vi "DAQ_PID_Actuator.vi"() -> ()   [LabVIEW 2019]
uses:
  <vilib>/Platform/TimedLoop/XDataNode/timing_clust.ctl
  <vilib>/Platform/TimedLoop/XDataNode/nitl_modes.ctl
  <vilib>/Platform/TimedLoop/XDataNode/wakeup.ctl
  <vilib>/Analysis/6fits.llb/Curve Fitting Criteria.ctl
  <vilib>/Analysis/3filter.llb/Filter Passband Type.ctl
  <vilib>/DAQmx/write.llb/DAQmx Write (Analog Wfm 1Chan NSamp).vi
  <vilib>/DAQmx/read.llb/DAQmx Read (Analog Wfm 1Chan NSamp).vi
  <vilib>/Analysis/baseanly.llb/Mean (DBL).vi
  <vilib>/Analysis/5stat.llb/RMS (DBL).vi
  <vilib>/DAQmx/create/channels.llb/DAQmx Create Channel (AO-Voltage-Basic).vi
  <vilib>/DAQmx/configure/timing.llb/DAQmx Timing (Sample Clock).vi
  <vilib>/DAQmx/miscellaneous.llb/DAQmx Fill In Error Info.vi
  <vilib>/DAQmx/create/channels.llb/DAQmx Create Channel (AI-Voltage-Basic).vi
  <vilib>/measure/mascope.llb/Amplitude and Levels 1 chan (obs).vi
  <vilib>/gmath/NumericalOptimization/Nonlinear Curve Fit LM formula string.vi
  <vilib>/platform/TimedLoop/XDataNode/XDataNode.xnode
  <vilib>/Analysis/NI_AALBase.lvlib
  <vilib>/Platform/TimedLoop/XDataNode/XDNodeRunTimeDep.lvlib
  <vilib>/gmath/NI_Gmath.lvlib
  <vilib>/Analysis/NI_AALPro.lvlib
  <vilib>/measure/NI_MABase.lvlib
  <vilib>/measure/NI_MAPro.lvlib
  <vilib>/ptbypt/NI_PtbyPt.lvlib
panel:
  out "Value":dbl min=-5.0 max=5.0 step=0.0001
  in  "Set Point Offset":dbl(slide) min=-5.0 max=5.0 step=0.0001 scale=-5.0..5.0
  in  "guessVoltage":dbl format="%#_13g"
  in  "PHASE":dbl format="%#_13g"
  in  "STOP":bool
  out "In Range?":bool=TRUE
  out "ELEMENT":dbl=0.9799129199459758
  in  "Ki":dbl=0.07
  in  "Kp":dbl=0.03
  out "SLOPE":dbl=-6.141102048812741
  out "OFFSET":dbl=1.2218182454508948
  out "Waveform Chart":dynamicdata(graph)=[{"t0"=timestamp(3637842565.871356 s since 1904-01-01), "dt"=1.0, "Y"=[2.0218377698329277]}, {"t0"=timestamp(3637842565.8663554 s since 1904-01-01), "dt"=1.0, "Y"=[0.25417959292529346]}, {"t0"=timestamp(3637842565.871356 s since 1904-01-01), "dt"=1.0, "Y"=[1.729518885187998]}, {"t0"=timestamp(3637842565.871356 s since 1904-01-01), "dt"=1.0, "Y"=[1.7676581769076343]}]
  in  "stop":bool
  out "Scanning":waveform(dbl)[](graph)=[{"t0"=timestamp(0 s since 1904-01-01), "dt"=0.000333325, "Y"=array[3000 elements]}, {"t0"=timestamp(0 s since 1904-01-01), "dt"=0.0003333333333333333, "Y"=array[3000 elements]}, {"t0"=timestamp(0 s since 1904-01-01), "dt"=0.000333325, "Y"=array[3000 elements], "attributes"=variant("NI_ChannelName"=variant(string "Filtered (Filtered)"), "NI_OriginalChannelName"=variant(string "Filtered"))}]
  in  "stop Lock":bool
  out "Locking":cluster{"Y":dbl[], "best nonlinear fit":dbl[]}[](graph)=[{"Y"=[1.5391142076213253], "best nonlinear fit"=[0.25417959292529346]}, {"Y"=array[214 elements], "best nonlinear fit"=array[214 elements]}, {"Y"=array[214 elements], "best nonlinear fit"=array[214 elements]}]
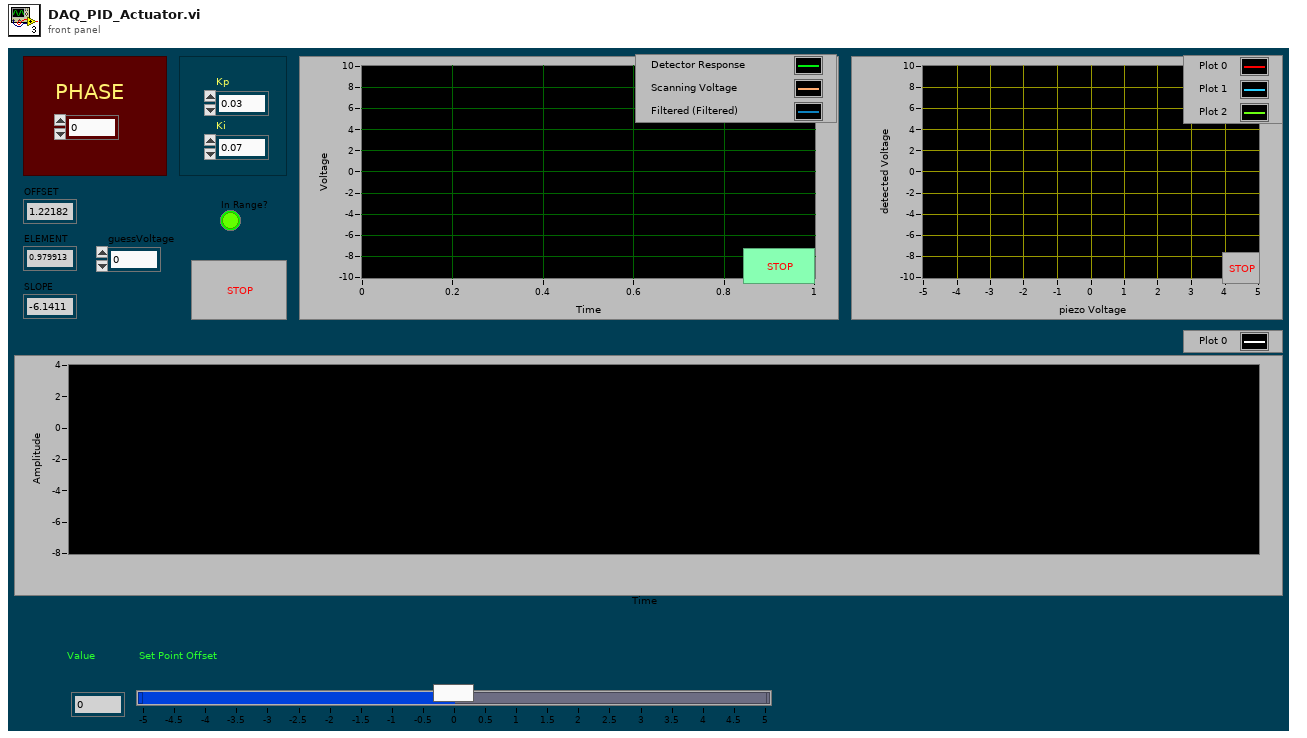
[diagram p1: front panel]
types:
  T1 = enum16{"Sine Wave", "Triangle Wave", "Square Wave", "Sawtooth Wave"}
  T2 = typedef "XDNodeRunTimeDep.lvlib/timing_clust.ctl" = cluster{"Expected End [f-1]":u64, "Actual End [f-1]":u64, "Finished Late? [f-1]":bool, "Expected End [i-1]":u64, "Actual End [i-1]":u64, "Finished Late? [i-1]":bool, "Expected Start [i]":u64, "Actual Start [i]":u64, "Expected Start [f]":u64, "Actual Start [f]":u64, "Source Name":string, "Structure Name":string, "Period":i64, "Deadline":i64, "Offset":i64, "Start":i64, "Priority":i32, "Timeout":i32, "Mode":T3, "Wakeup Reason":T4, "Error":errorcluster, "Source Type":string, "Secondary Source Type":string, "Global End Time":u64, "Global Start Time":u64, "Frame Duration":u64, "Iteration Duration":u64, "Assigned CPU":i32, "I/O Scan Engine Mode":u32}
  T3 = typedef "XDNodeRunTimeDep.lvlib/nitl_modes.ctl" = enum32{"No Change", "Process missed periods, maintain original phase", "Discard missed periods, maintain original phase", "Process missed periods, ignore original phase", "Discard missed periods, ignore original phase"}
  T4 = typedef "XDNodeRunTimeDep.lvlib/wakeup.ctl" = enum32{"Normal", "Aborted", "Asynchronous wakeup", "Timing source error", "Timed loop error", "Timeout"}
  T5 = cluster{"slope min":dbl, "slope max":dbl, "intercept min":dbl, "intercept max":dbl}
  T6 = cluster{"model":string, "Parameters":string[], "x":string}
  T7 = enum16{"arithmetic", "geometric", "harmonic", "trimmed", "median"}
  T8 = typedef "NI_AALBase.lvlib/Filter Passband Type.ctl" = enum32{"Lowpass", "Highpass", "Bandpass", "Bandstop"}
  T9 = typedef "NI_AALPro.lvlib/Curve Fitting Criteria.ctl" = u16
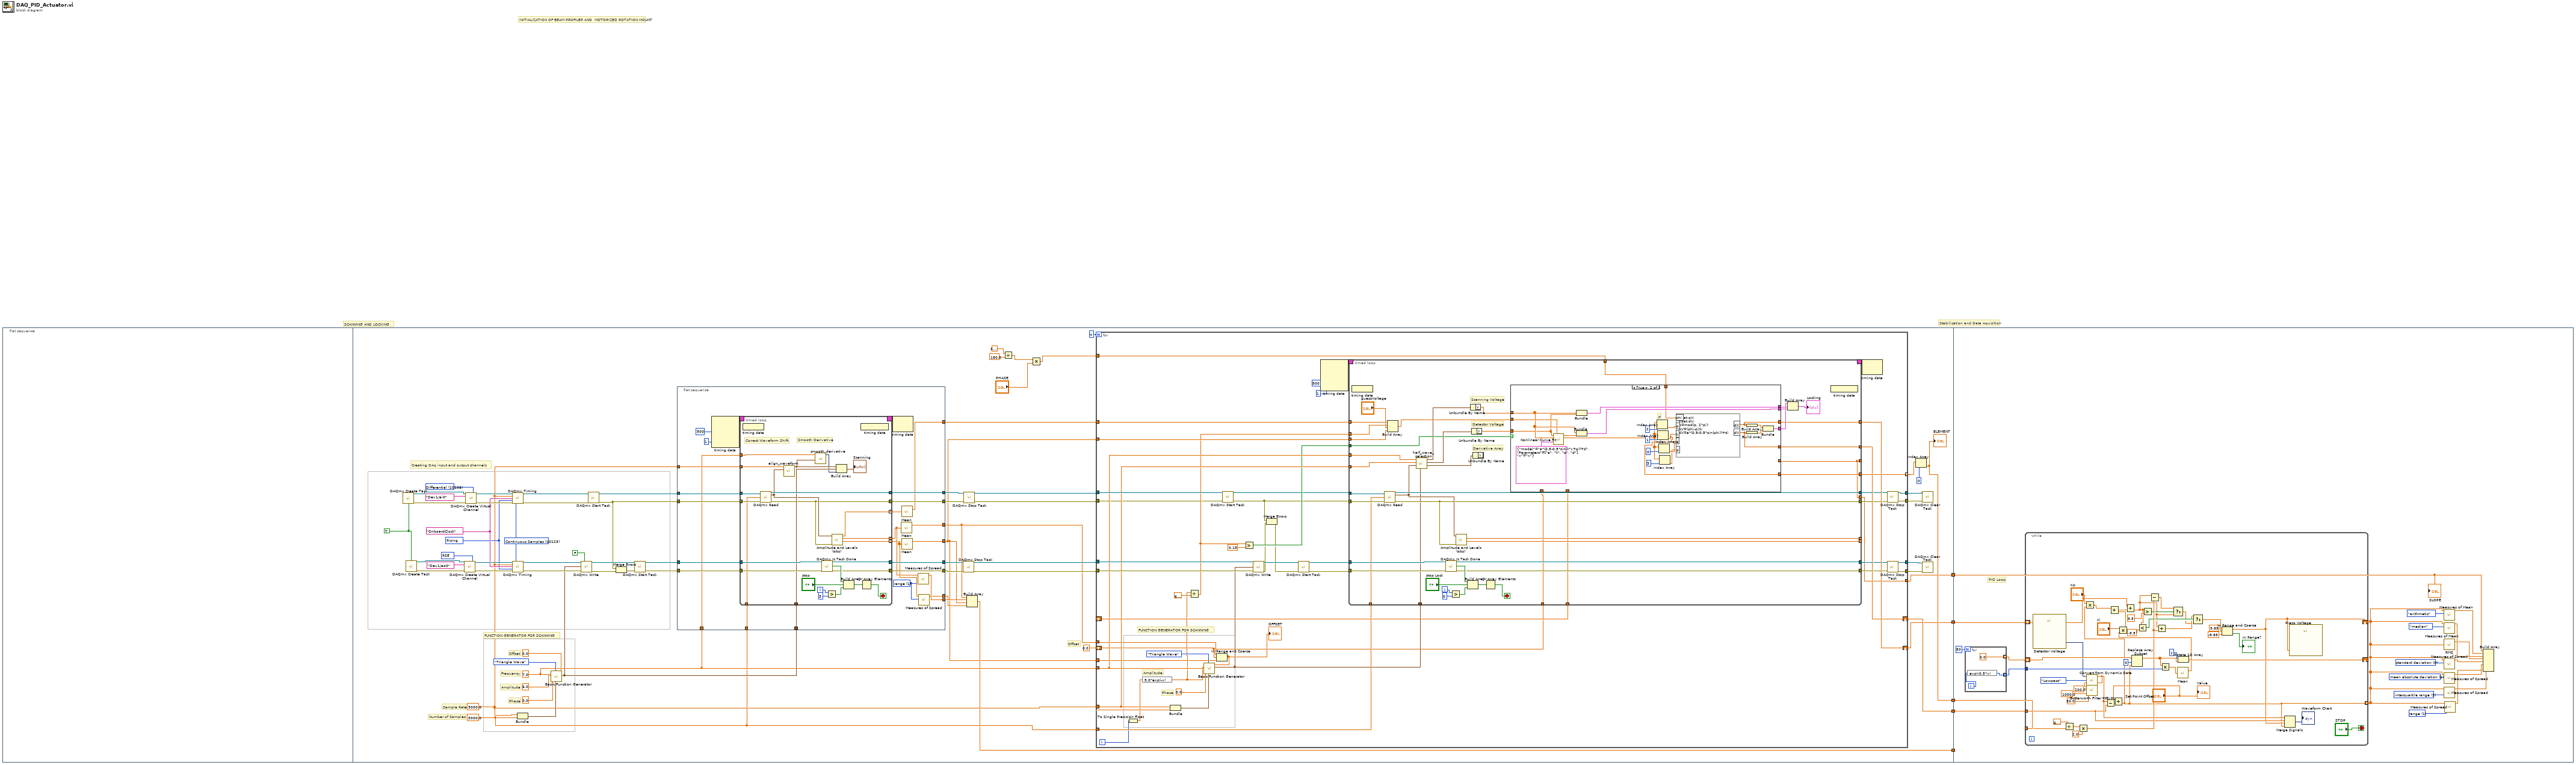
[diagram p0: block diagram]
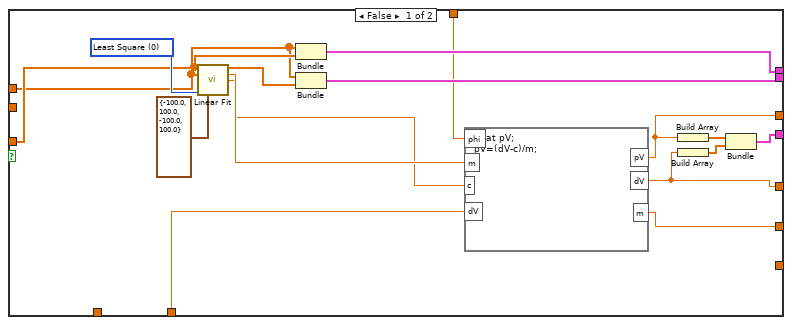
[diagram p2: hidden frame]
diagram:
  # "Stabilization and Data Aquisition"
  # "SCANNING AND LOCKING"
  # "INITIALIZATION OF BEAM PROFILER AND  MOTORIZED ROTATION MOUNT"
  n1 = flat-sequence {
    tunnel: [w21] -> w5
    tunnel: [w18] -> w4
    tunnel: [w17] -> w3
    tunnel: [w14] -> w2
    tunnel: [w13] -> w1
    tunnel: w5 -> [w291]
    tunnel: w4 -> [_]
    tunnel: w3 -> [w277]
    tunnel: w2 -> [w272]
    tunnel: w1 -> [w271]
    frame #0 {
    }
    frame #1 {
      w37 = TRUE ("auto cleanup")
      w23 = 3000.0
      w24 = 7.0 ("frequency")
      w63 = 10123 items=["Finite Samples"=10178, "Continuous Samples"=10123, "Hardware Timed Single Point"=12522] ("sample mode")
      w22 = 3000.0
      w64 = 10280 items=["Rising"=10280, "Falling"=10171] ("active edge")
      w69 = tag "OnboardClock" ("source")
      w70 = 10083 items=["Default"=-1, "RSE"=10083, "Differential"=10106, "Pseudodifferential"=12529] ("output terminal configuration")
      w72 = 10106 items=["Default"=-1, "RSE"=10083, "NRSE"=10078, "Differential"=10106, "Pseudodifferential"=12529] ("input terminal configuration")
      # "Number of Samples"
      # "FUNCTION GENERATOR FOR SCANNING"
      # "Phase"
      # "Amplitude"
      # "Frequency"
      # "Offset"
      # "Sample Rate"
      # "Creating DAq input and output channels"
      # "Offset"
      n2 = call <vilib>:"DAQmx Create Task.vi"("auto cleanup"=w37) -> ("task out"=w40:refnum<k21>, "error out"=w39:errorcluster)  [unwired: 13 in]
      n3 = call <vilib>:"DAQmx Create Task.vi"("auto cleanup"=w37) -> ("task out"=w38:refnum<k21>, "error out"=w36:errorcluster)  [unwired: 13 in]
      n4 = call-poly <vilib>:"DAQmx Create Virtual Channel.vi"("task in"=w38, "output terminal configuration"=w70, "physical channels"=tag "Dev1/ao0", "error in"=w36) -> ("task out"=w66:refnum<k21>, "error out"=w65:errorcluster)  [unwired: 10 in]
      n5 = call-poly <vilib>:"DAQmx Create Virtual Channel.vi"("task in"=w40, "input terminal configuration"=w72, "physical channels"=tag "Dev1/ai0", "error in"=w39) -> ("task out"=w68:refnum<k21>, "error out"=w67:errorcluster)  [unwired: 10 in]
      n6 = call-poly <vilib>:"DAQmx Timing.vi"("task/channels in"=w68, "sample mode"=w63, "rate"=w22, "source"=w69, "active edge"=w64, "error in"=w67) -> ("task out"=w54:refnum<k21>, "error out"=w53:errorcluster)  [unwired: 8 in]
      n7 = call-poly <vilib>:"DAQmx Timing.vi"("task/channels in"=w66, "sample mode"=w63, "rate"=w22, "source"=w69, "active edge"=w64, "error in"=w65) -> ("task out"=w62:refnum<k21>, "error out"=w61:errorcluster)  [unwired: 8 in]
      n8 = Bundle(w22, w23) -> (w56:cluster{dbl, dbl})  [unwired: 1 in]
      n9 = call <vilib>:"Basic Function Generator.vi"("offset"=0.0, "sampling info"=w56, "signal type"=T1."Triangle Wave", "phase"=0.0, "amplitude"=6.0, "frequency"=w24) -> ("signal out"=w51:waveform(dbl))  [unwired: 3 in, 2 out]
      n10 = call-poly <vilib>:"DAQmx Write.vi"("task/channels in"=w62, "auto start"=FALSE, "data"=w51, "error in"=w61) -> ("task out"=w55:refnum<k21>, "error out"=w46:errorcluster)  [unwired: 9 in, 1 out]
      n11 = call <vilib>:"DAQmx Start Task.vi"("task/channels in"=w54, "error in"=w53) -> ("task out"=w52:refnum<k21>, "error out"=w47:errorcluster)  [unwired: 12 in]
      n12 = Merge Errors(w47, w46) -> (w48:errorcluster)
      n13 = call <vilib>:"DAQmx Start Task.vi"("task/channels in"=w55, "error in"=w48) -> ("task out"=w49:refnum<k21>, "error out"=w50:errorcluster)  [unwired: 12 in]
      n14 = flat-sequence {
        tunnel: w52 -> [w96]
        tunnel: w47 -> [w95]
        tunnel: w51 -> [w94]
        tunnel: w50 -> [w93]
        tunnel: w49 -> [w92]
        tunnel: w22 -> [w90]
        tunnel: w23 -> [w89]
        tunnel: w24 -> [w88]
        tunnel: [w87] -> w42
        tunnel: [w86] -> w44
        tunnel: [w85] -> w43
        tunnel: [w84] -> w41
        tunnel: [w82] -> w27
        tunnel: [w81] -> w12
        tunnel: [w80] -> w11
        tunnel: [w75] -> w20
        tunnel: [w74] -> w19
        frame #0 {
          w76 = 1 items=["standard deviation", "range", "mean absolute deviation", "interquartile range"] ("type")
          n15 = node-c288(i64 500 ("Period"), 1 ("Processor")) -> (w98:T2)  [unwired: 2 in]
          n16 = timed-loop {
            timing: w98 -> [_]
            timing-out: [_] -> w97
            tunnel: w96 -> [w124]
            tunnel: w95 -> [w123]
            tunnel: w94 -> [w109]
            tunnel: w93 -> [w112]
            tunnel: w92 -> [w122]
            tunnel: [w114] -> w87
            tunnel: [w103] -> w84
            tunnel: [w113] -> w86
            tunnel: [w111] -> w85
            tunnel: w90 -> [w108]
            tunnel: w89 -> [w107]
            tunnel: w88 -> [w105]
            tunnel: [w102] -> w78 mode=indexing
            tunnel: [w101] -> w77 mode=indexing
            tunnel: [w100] -> w83 mode=indexing
            i -> [w119]
            stop <- w115 stop-if-true
            # "Smooth Derivative"
            # "Correct Waveform Shift"
            n17 = node-c288() -> ()  [unwired: 1 in]
            n18 = call-poly <vilib>:"DAQmx Read.vi"("task/channels in"=w124, "number of samples per channel"=w107, "error in"=w123) -> ("task out"=w114:refnum<k21>, "data"=w104:waveform(dbl), "error out"=w103:errorcluster)  [unwired: 10 in]
            n19 = call "align_waveform.vi"("Input Waveform"=w104, "Sample Rate to be Wired"=w108) -> ("Output Waveform"=w106:waveform(dbl))  [unwired: 9 in]
            n20 = call "smooth_derivative.vi"("Output Waveform"=w106, "frequency"=w105) -> ("Filtered Signal"=w99:dynamicdata)  [unwired: 9 in]
            n21 = call <vilib>:"DAQmx Is Task Done.vi"("task/channels in"=w122, "error in"=w112) -> ("task out"=w113:refnum<k21>, "task done?"=w120:bool, "error out"=w111:errorcluster)  [unwired: 11 in]
            n22 = Greater?(x=w119, y=3) -> (0:w116:bool)
            n23 = call-poly <vilib>:"Amplitude and Levels (obs).vi"("error in (no error)"=w103, "signal in"=w104) -> ("low state level"=w101:dbl, "high state level"=w102:dbl, "amplitude"=w100:dbl)  [unwired: 6 in, 1 out]
            n24 = Build Array(w106, w109, w99) -> (→"Scanning":waveform(dbl)[])
            n25 = Build Array(w120, "stop", w116) -> (w121:bool[])
            n26 = node-c288() -> ()  [unwired: 1 out]
            n27 = Or Array Elements(Boolean array=w121) -> (logical OR=w115:bool)
          }
          n28 = node-c288(w97) -> ()  [unwired: 1 out]
          n29 = call-poly <vilib>:"Mean.vi"("X"=w78) -> ("mean"=w81:dbl)  [unwired: 1 out]
          n30 = call-poly <vilib>:"Mean.vi"("X"=w83) -> ("mean"=w82:dbl)  [unwired: 1 out]
          n31 = call-poly <vilib>:"Mean.vi"("X"=w77) -> ("mean"=w80:dbl)  [unwired: 1 out]
          n32 = call <vilib>:"Measures of Spread.vi"("type"=w76, "x array"=w78) -> ("spread value"=w75:dbl)  [unwired: 8 in, 1 out]
          n33 = call <vilib>:"Measures of Spread.vi"("type"=w76, "x array"=w77) -> ("spread value"=w74:dbl)  [unwired: 8 in, 1 out]
        }
      }
      n34 = call <vilib>:"DAQmx Stop Task.vi"("task/channels in"=w44, "error in"=w43) -> ("task out"=w26:refnum<k21>, "error out"=w25:errorcluster)  [unwired: 12 in]
      n35 = call <vilib>:"DAQmx Stop Task.vi"("task/channels in"=w42, "error in"=w41) -> ("task out"=w29:refnum<k21>, "error out"=w28:errorcluster)  [unwired: 12 in]
      n36 = Build Array(w12, w20, w11, w19) -> (w18:dbl[])
      n37 = Divide(x=3.141592653589793, y=180.0) -> (x/y=w10:dbl)
      n38 = Multiply(x=w10, y="PHASE") -> (x*y=w6:dbl)
      n39 = for {
        N: 4 -> [_]
        tunnel: w23 -> [w172]
        tunnel: w24 -> [w170]
        tunnel: w22 -> [w169]
        tunnel: w27 -> [w168]
        tunnel: w11 -> [w167]
        tunnel: w29 -> [w171]
        tunnel: w28 -> [w147]
        tunnel: w26 -> [w178]
        tunnel: w25 -> [w177]
        shift-right: [w162] -> w13
        shift-left: 0.0 ("offset") -> [w136]
        shift-right: [w156] -> w21
        shift-left: _ -> [w155]
        tunnel: [w144] -> w31
        tunnel: [w143] -> w30
        tunnel: [w140] -> w33
        tunnel: [w139] -> w32
        tunnel: [w138] -> w16 mode=indexing
        tunnel: [w137] -> w14
        tunnel: w12 -> [w135]
        tunnel: w11 -> [w134]
        tunnel: w6 -> [w132]
        i -> [w164]
        # "FUNCTION GENERATOR FOR SCANNING"
        # "Phase"
        # "Amplitude"
        n40 = To Single Precision Float(number=w164) -> (single precision float=w163:sgl)
        n41 = expression code="5.0*exp(-x)"(w163) -> (w165:sgl)
        n42 = Bundle(w169, w172) -> (w174:cluster{dbl, dbl})  [unwired: 1 in]
        n43 = Divide(x=w165, y=6.283185307179586) -> (x/y=w159:dbl)
        n44 = In Range and Coerce(upper limit=w135, x=w136, lower limit=w134) -> (coerced(x)=w133:dbl)  [unwired: 1 out]
        "OFFSET" <- w133
        n45 = call <vilib>:"Basic Function Generator.vi"("offset"=w133, "sampling info"=w174, "signal type"=T1."Triangle Wave", "phase"=0.0, "amplitude"=w165, "frequency"=w170) -> ("signal out"=w173:waveform(dbl))  [unwired: 3 in, 2 out]
        n46 = call <vilib>:"DAQmx Start Task.vi"("task/channels in"=w171, "error in"=w147) -> ("task out"=w149:refnum<k21>, "error out"=w148:errorcluster)  [unwired: 12 in]
        n47 = Greater?(x=w159, y=0.15) -> (0:w157:bool)
        n48 = call-poly <vilib>:"DAQmx Write.vi"("task/channels in"=w178, "data"=w173, "error in"=w177) -> ("task out"=w152:refnum<k21>, "error out"=w151:errorcluster)  [unwired: 10 in, 1 out]
        n49 = Merge Errors(w148, w151) -> (w150:errorcluster)
        n50 = call <vilib>:"DAQmx Start Task.vi"("task/channels in"=w152, "error in"=w150) -> ("task out"=w154:refnum<k21>, "error out"=w153:errorcluster)  [unwired: 12 in]
        n51 = node-c288(i64 500 ("Period"), 1 ("Processor")) -> (w180:T2)  [unwired: 2 in]
        n52 = timed-loop {
          timing: w180 -> [_]
          timing-out: [_] -> w179
          tunnel: w149 -> [w224]
          tunnel: w148 -> [w223]
          tunnel: w173 -> [w203]
          tunnel: w153 -> [w212]
          tunnel: w154 -> [w222]
          tunnel: [w214] -> w142
          tunnel: [w208] -> w141
          tunnel: [w213] -> w146
          tunnel: [w211] -> w145
          tunnel: w169 -> [w205]
          tunnel: w172 -> [w210]
          tunnel: w170 -> [w204]
          tunnel: [w207] -> _ mode=indexing
          tunnel: [w206] -> _ mode=indexing
          tunnel: w168 -> [w199]
          tunnel: w167 -> [w190]
          tunnel: w159 -> [w198]
          tunnel: [w188] -> w162
          tunnel: w157 -> [w187]
          tunnel: w136 -> [w186]
          tunnel: [w185] -> w156
          tunnel: w155 -> [w184]
          tunnel: [w183] -> w138
          tunnel: [w182] -> _
          tunnel: [w182] -> w137
          tunnel: w132 -> [w181]
          i -> [w219]
          stop <- w215 stop-if-true
          # "Derivative Array"
          # "Detector Voltage"
          # "Scanning Voltage"
          n53 = node-c288() -> ()  [unwired: 1 in]
          n54 = call-poly <vilib>:"DAQmx Read.vi"("task/channels in"=w224, "number of samples per channel"=w210, "error in"=w223) -> ("task out"=w214:refnum<k21>, "data"=w209:waveform(dbl), "error out"=w208:errorcluster)  [unwired: 10 in]
          n55 = Build Array(w199, w198, "guessVoltage", w190) -> (w197:dbl[])
          n56 = call "half_wave_selection.vi"("signal in"=w203, "data"=w209, "Numeric"=w205, "frequency"=w204) -> ("waveform out"=w200:waveform(dbl), "waveform out 2"=w201:waveform(dbl), "waveform out 3"=w202:waveform(dbl))  [unwired: 5 in]
          n57 = call <vilib>:"DAQmx Is Task Done.vi"("task/channels in"=w222, "error in"=w212) -> ("task out"=w213:refnum<k21>, "task done?"=w220:bool, "error out"=w211:errorcluster)  [unwired: 11 in]
          n58 = Greater?(x=w219, y=0) -> (0:w216:bool)
          n59 = call-poly <vilib>:"Amplitude and Levels (obs).vi"("error in (no error)"=w208, "signal in"=w209) -> ("low state level"=w206:dbl, "high state level"=w207:dbl)  [unwired: 6 in, 2 out]
          n60 = Build Array(w220, "stop Lock", w216) -> (w221:bool[])
          n61 = Unbundle By Name(w202) -> ("Y"=w196:dbl[])
          n62 = Unbundle By Name(w201) -> ("Y"=w195:dbl[])
          n63 = Unbundle By Name(w200) -> ()  [unwired: 1 out]
          n64 = Or Array Elements(Boolean array=w221) -> (logical OR=w215:bool)
          n65 = case shown="True" w187 {
            tunnel: w197 -> [_ w262]
            tunnel: w196 -> [w237 w260]
            tunnel: w195 -> [w239 w259]
            tunnel: [w238 w258] -> w194
            tunnel: [w235 w257] -> w193
            tunnel: w181 -> [w233 w256]
            tunnel: [w229 w246] -> w189
            tunnel: [w226 w245] -> w188
            tunnel: w186 -> [_ _]
            tunnel: [w227 w244] -> w185
            tunnel: w184 -> [w230 _]
            tunnel: [_ w242] -> w183
            tunnel: [w225 _] -> w182
            frame False {
              w241 = T9 0 items=["Least Square", "Least Absolute Residual", "Bisquare"] ("method")
              n66 = call <vilib>:"Linear Fit.vi"("Y"=w239, "X"=w237, "method"=w241, "parameter bounds"=T5 {"slope min"=-100.0, "slope max"=100.0, "intercept min"=-100.0, "intercept max"=100.0}) -> ("Best Linear Fit"=w236:dbl[], "slope"=w232:dbl, "intercept"=w231:dbl)  [unwired: 7 in, 2 out]
              n67 = Bundle("Y"=w237, "Y"=w239) -> (w238:cluster{"Y":dbl[], "Y":dbl[]})  [unwired: 1 in]
              n68 = Bundle("Y"=w237, "Best Linear Fit"=w236) -> (w235:cluster{"Y":dbl[], "Best Linear Fit":dbl[]})  [unwired: 1 in]
              n69 = formula code="float pV;\npV=(dV-c)/m;"("phi"=w233, "m"=w232, "c"=w231, "dV"=w230) -> ("pV"=w226:dbl, "dV"=w227:dbl, "m"=w225:dbl)
              n70 = Build Array(w226) -> (w228:dbl[])
              n71 = Build Array(w227) -> (w234:dbl[])
              n72 = Bundle(w228, w234) -> (w229:cluster{dbl[], dbl[]})  [unwired: 1 in]
            }
            frame True {
              # "p"
              n73 = call-poly <vilib>:"Nonlinear Curve Fit.vi"("Y"=w259, "initial parameters"=w262, "X"=w260, "model description"=T6 {"model"="a*(0.5-0.5*sin(k*x+p))+d", "Parameters"=["a", "k", "p", "d"], "x"="x"}) -> ("best nonlinear fit"=w261:dbl[], "best fit parameters"=w250:dbl[])  [unwired: 7 in, 3 out]
              n74 = Bundle("Y"=w260, "Y"=w259) -> (w258:cluster{"Y":dbl[], "Y":dbl[]})  [unwired: 1 in]
              n75 = Bundle("Y"=w260, "best nonlinear fit"=w261) -> (w257:cluster{"Y":dbl[], "best nonlinear fit":dbl[]})  [unwired: 1 in]
              n76 = Index Array(array=w250, index=2) -> (element=w253:dbl)
              n77 = Index Array(array=w250, index=1) -> (element=w242:dbl)
              n78 = Index Array(array=w250, index=0) -> (element=w252:dbl)
              n79 = Index Array(array=w250, index=3) -> (element=w243:dbl)
              n80 = formula code="float pV;\nfloat dV;\np=mod(p, 2*pi);\npV=(phi-p)/k;\ndV=a*(0.5-0.5*sin(phi))+d;"("phi"=w256, "p"=w253, "k"=w242, "a"=w252, "d"=w243) -> ("pV"=w245:dbl, "dV"=w244:dbl)
              n81 = Build Array(w245) -> (w248:dbl[])
              n82 = Build Array(w244) -> (w247:dbl[])
              n83 = Bundle(w248, w247) -> (w246:cluster{dbl[], dbl[]})  [unwired: 1 in]
            }
          }
          n84 = Build Array(w189, w194, w193) -> (→"Locking":cluster{"Y":dbl[], "best nonlinear fit":dbl[]}[])
          n85 = node-c288() -> ()  [unwired: 1 out]
        }
        n86 = node-c288(w179) -> ()  [unwired: 1 out]
        n87 = call <vilib>:"DAQmx Stop Task.vi"("task/channels in"=w142, "error in"=w141) -> ("task out"=w140:refnum<k21>, "error out"=w139:errorcluster)  [unwired: 12 in]
        n88 = call <vilib>:"DAQmx Stop Task.vi"("task/channels in"=w146, "error in"=w145) -> ("task out"=w144:refnum<k21>, "error out"=w143:errorcluster)  [unwired: 12 in]
      }
      n89 = Index Array(array=w16, index=0) -> (element=w17:dbl)
      "ELEMENT" <- w17
      n90 = call <vilib>:"DAQmx Clear Task.vi"("task in"=w33, "error in"=w32) -> ()  [unwired: 13 in, 1 out]
      n91 = call <vilib>:"DAQmx Clear Task.vi"("task in"=w31, "error in"=w30) -> ()  [unwired: 13 in, 1 out]
    }
    frame #2 {
      w287 = 0 items=["standard deviation", "range", "mean absolute deviation", "interquartile range"] ("type")
      w288 = 2 items=["standard deviation", "range", "mean absolute deviation", "interquartile range"] ("type")
      w289 = 3 items=["standard deviation", "range", "mean absolute deviation", "interquartile range"] ("type")
      w290 = 1 items=["standard deviation", "range", "mean absolute deviation", "interquartile range"] ("type")
      # "PID Loop"
      n92 = for {
        N: 50 -> [_]
        tunnel: [w337] -> w274 mode=indexing
        tunnel: [0.0] -> w275 mode=indexing
        i -> [w338]
        n93 = expression code="exp(-0.5*x)"(w338) -> (w337:i32)
      }
      n94 = while {
        tunnel: w291 -> [w301]
        tunnel: w277 -> [w334]
        shift-right: [w327] -> _
        shift-left: w275 -> [w330]
        tunnel: w274 -> [w325]
        tunnel: [w293] -> w273 mode=indexing
        shift-right: [w300] -> _
        shift-left: w271 -> [w308]
        stop <- "STOP" stop-if-true
        n95 = call "Detector Voltage"() -> ("data"=w323:dynamicdata)  [unwired: 17 in, 2 out]
        n96 = Divide(x=6.283185307179586, y=w334) -> (x/y=w332:dbl)
        n97 = Multiply(x=w332, y=2.0) -> (x*y=w317:dbl)
        n98 = call "Convert from Dynamic Data"("Dynamic Data Type"=w323) -> ("Scalar"=w297:dbl)  [unwired: 3 in]
        n99 = call <vilib>:"Butterworth Filter PtByPt.vi"("filter type"=Filter_Passband_Type."Lowpass", "low cutoff freq: fl"=50.0, "high cutoff freq: fh"=1000.0, "sampling freq: fs"=200.0, "x"=w297) -> ()  [unwired: 4 in, 2 out]
        n100 = Subtract(x=w297, y=w301) -> (x-y=w299:dbl)
        n101 = Add(x="Set Point Offset", y=w299) -> (x+y=w293:dbl)
        n102 = Multiply(x="Kp", y=w293) -> (x*y=w319:dbl)
        n103 = Replace Array Subset(array=w330, new element=w293, index=0) -> (w326:dbl[])
        n104 = Multiply(x=w326, y=w325) -> (x*y=w324:dbl[])
        n105 = call-poly <vilib>:"Mean.vi"("X"=w324) -> ("mean"=w320:dbl)  [unwired: 1 out]
        n106 = Multiply(x="Ki", y=w320) -> (x*y=w318:dbl)
        n107 = Add(x=w319, y=w318) -> (x+y=w313:dbl)
        n108 = Add(x=w308, y=w313) -> (x+y=w309:dbl)
        n109 = Less?(x=w309, y=-9.5) -> (x < y?=w312:bool)
        n110 = Greater?(x=w309, y=9.5) -> (0:w316:bool)
        n111 = Subtract(x=w309, y=w317) -> (x-y=w315:dbl)
        n112 = Add(x=w309, y=w317) -> (x+y=w311:dbl)
        n113 = Select(t=w315, s=w316, f=w309) -> (s? t:f=w310:dbl)
        n114 = Rotate 1D Array(1:w326, 2:1 ("n")) -> (0:w327:dbl[])
        n115 = Select(t=w311, s=w312, f=w310) -> (s? t:f=w306:dbl)
        n116 = In Range and Coerce(upper limit=9.85, x=w306, lower limit=-9.85) -> (coerced(x)=w300:dbl, In Range?=→"In Range?":bool)
        n117 = Merge Signals(w297, w301, w300, w293) -> (→"Waveform Chart":dynamicdata)
        n118 = call "Piezo Voltage"("data"=w300) -> ()  [unwired: 17 in, 2 out]
        "Value" <- "Set Point Offset"
      }
      n119 = call <vilib>:"Measures of Mean.vi"("type"=T7."arithmetic", "x array"=w273) -> ("mean value"=w284:dbl)  [unwired: 8 in, 1 out]
      n120 = call <vilib>:"Measures of Mean.vi"("type"=T7."median", "x array"=w273) -> ("mean value"=w283:dbl)  [unwired: 8 in, 1 out]
      n121 = call <vilib>:"Measures of Spread.vi"("type"=w288, "x array"=w273) -> ("spread value"=w280:dbl)  [unwired: 8 in, 1 out]
      n122 = call <vilib>:"Measures of Spread.vi"("type"=w289, "x array"=w273) -> ("spread value"=w279:dbl)  [unwired: 8 in, 1 out]
      n123 = call-poly <vilib>:"RMS.vi"("X"=w273) -> ("rms value"=w282:dbl)  [unwired: 1 out]
      n124 = call <vilib>:"Measures of Spread.vi"("type"=w287, "x array"=w273) -> ("spread value"=w281:dbl)  [unwired: 8 in, 1 out]
      n125 = call <vilib>:"Measures of Spread.vi"("type"=w290, "x array"=w273) -> ("spread value"=w278:dbl)  [unwired: 8 in, 1 out]
      n126 = Build Array(w272, w284, w283, w282, w281, w280, w279, w278) -> ()  [unwired: 1 out]
      "SLOPE" <- w272
    }
  }
